vi "Odbior danych z PC .vi"(8 "error in (no error)":errorcluster, 11 "connection ID":refnum<k16>) -> (0 "error out":errorcluster, 3 "connection ID out":refnum<k16>, 5 "Output Data":T1)   [LabVIEW 2015]
uses:
  PC/QMH Fundamentals - Message Cluster.ctl
  <vilib>/RioEmbeddedCAN/RioEmbeddedCAN.llb/CANFrameControl.ctl
  safety_ctl.ctl
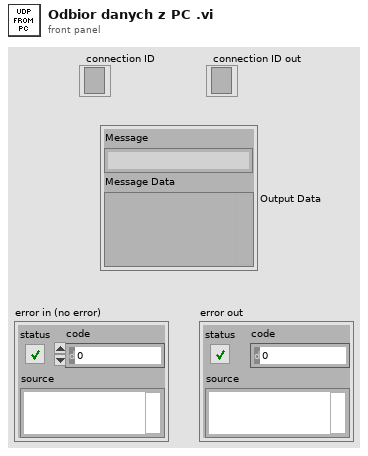
[diagram p1: front panel]
types:
  T1 = typedef "QMH Fundamentals - Message Cluster.ctl" = cluster{"Message":string, "Message Data":variant}
  T2 = cluster{"Data":cluster{"date/time string":string, "array of cans":cluster{"identifier":u32, "extended?":bool, "type":u8, "payload":u8[]}[]}, "bool":bool}
  T3 = cluster{"date/time string":string, "array of cans":cluster{"identifier":u32, "extended?":bool, "type":u8, "payload":u8[]}[]}
  T4 = typedef "CANFrameControl.ctl" = cluster{"identifier":u32, "extended?":bool, "type":u8, "payload":u8[]}
  T5 = cluster{"PITCH 1":dbl, "YAW 1":dbl, "ROLL 1":dbl}
  T6 = cluster{"bool":bool, "Gimbale":cluster{"PITCH 1":dbl, "YAW 1":dbl, "ROLL 1":dbl}}
  T7 = typedef "safety_ctl.ctl" = cluster{"reset_stm":bool, "stop":bool}
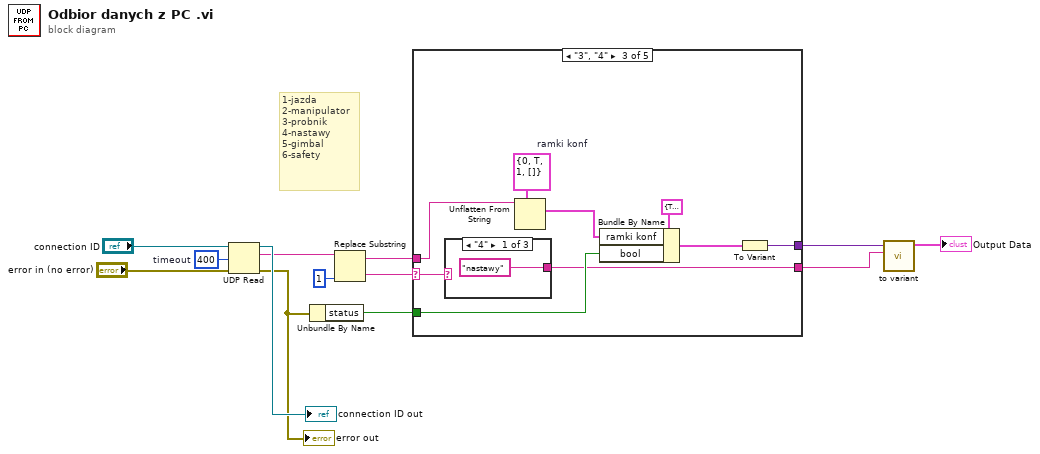
[diagram p0: block diagram]
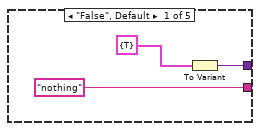
[diagram p2: hidden frame]
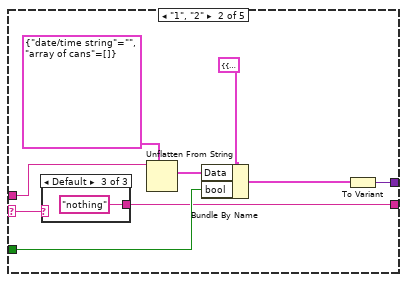
[diagram p3: hidden frame]
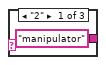
[diagram p4: hidden frame]
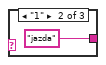
[diagram p5: hidden frame]
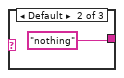
[diagram p6: hidden frame]
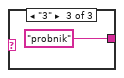
[diagram p7: hidden frame]
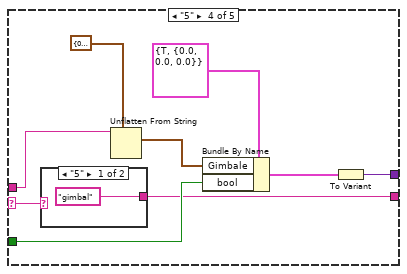
[diagram p8: hidden frame]
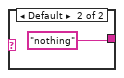
[diagram p9: hidden frame]
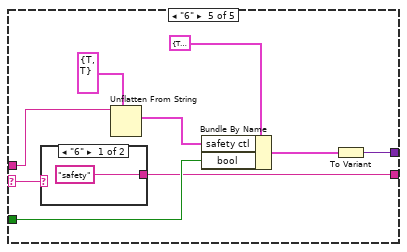
[diagram p10: hidden frame]
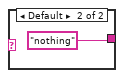
[diagram p11: hidden frame]
diagram:
  w11 = 400  # timeout
  # "1-jazda\n2-manipulator\n3-probnik\n4-nastawy\n5-gimbal\n6-safety"
  n1 = UDP Read(connection ID="connection ID", timeout ms (25000)=w11, 8:"error in (no error)") -> (data out=w8:string, error out=w5:errorcluster, 3:→"connection ID out":refnum<k16>)  [unwired: 1 in, 2 out]
  "error out" <- w5
  n2 = Unbundle By Name(w5) -> ("status"=w4:bool)
  n3 = Replace Substring(2:1 ("length (len. of substring)"), 5:w8) -> (0:w7:string, 1:w6:string)  [unwired: 2 in]
  n4 = case shown="\"3\", \"4\"" w7 {
    selector: w7 -> [_ w21 w35 w48 w59]
    tunnel: w6 -> [_ w24 w36 w49 w60]
    tunnel: w4 -> [_ w20 w32 w46 w57]
    tunnel: ["nothing" w19 w31 w45 w56] -> w2
    tunnel: [w15 w18 w29 w43 w54] -> w1
    frame "False", Default {
      n5 = To Variant(anything=cluster{bool} {TRUE}) -> (Variant=w15:variant)
    }
    frame "1", "2" {
      n6 = case shown="Default" w21 {
        tunnel: ["manipulator" "jazda" "nothing"] -> w19
        frame "2" {
        }
        frame "1" {
        }
        frame Default {
        }
      }
      n7 = Unflatten From String(type=T3 {"date/time string"="", "array of cans"=[]} ("output cluster"), binary string=w24) -> (value=w23:T3)  [unwired: 3 in, 2 out]
      n8 = Bundle By Name(cluster=T2 {"Data"={"date/time string"="", "array of cans"=[]}, "bool"=TRUE} ("jazda"), "Data"=w23, "bool"=w20) -> (w17:T2)
      n9 = To Variant(anything=w17) -> (Variant=w18:variant)
    }
    frame "3", "4" {
      w37 = T4 {"identifier"=0, "extended?"=TRUE, "type"=1, "payload"=[]}  # ramki konf
      n10 = case shown="\"4\"" w35 {
        tunnel: ["nastawy" "nothing" "probnik"] -> w31
        frame "4" {
        }
        frame Default {
        }
        frame "3" {
        }
      }
      n11 = Unflatten From String(type=w37, binary string=w36) -> (value=w33:T4)  [unwired: 3 in, 2 out]
      n12 = Bundle By Name(cluster=cluster{"bool":bool, "ramki konf":T4} {"bool"=TRUE, "ramki konf"={"identifier"=0, "extended?"=TRUE, "type"=1, "payload"=[]}} ("jazda"), "ramki konf"=w33, "bool"=w32) -> (w30:cluster{"bool":bool, "ramki konf":T4})
      n13 = To Variant(anything=w30) -> (Variant=w29:variant)
    }
    frame "5" {
      n14 = case shown="\"5\"" w48 {
        tunnel: ["gimbal" "nothing"] -> w45
        frame "5" {
        }
        frame Default {
        }
      }
      n15 = Unflatten From String(type=T5 {"PITCH 1"=0.0, "YAW 1"=0.0, "ROLL 1"=0.0} ("Gimbale"), binary string=w49) -> (value=w41:T5)  [unwired: 3 in, 2 out]
      n16 = Bundle By Name(cluster=T6 {"bool"=TRUE, "Gimbale"={"PITCH 1"=0.0, "YAW 1"=0.0, "ROLL 1"=0.0}} ("jazda"), "Gimbale"=w41, "bool"=w46) -> (w44:T6)
      n17 = To Variant(anything=w44) -> (Variant=w43:variant)
    }
    frame "6" {
      n18 = case shown="\"6\"" w59 {
        tunnel: ["safety" "nothing"] -> w56
        frame "6" {
        }
        frame Default {
        }
      }
      n19 = Unflatten From String(type=T7 {"reset_stm"=TRUE, "stop"=TRUE} ("safety ctl"), binary string=w60) -> (value=w53:T7)  [unwired: 3 in, 2 out]
      n20 = Bundle By Name(cluster=cluster{"bool":bool, "safety ctl":T7} {"bool"=TRUE, "safety ctl"={"reset_stm"=TRUE, "stop"=TRUE}} ("jazda"), "safety ctl"=w53, "bool"=w57) -> (w55:cluster{"bool":bool, "safety ctl":T7})
      n21 = To Variant(anything=w55) -> (Variant=w54:variant)
    }
  }
  n22 = call "to variant.vi"("Message"=w2, "Variant"=w1) -> ("Message Cluster"=→"Output Data":T1)  [unwired: 9 in]
